vi "Nested_Case_structure.vi"() -> ()   [LabVIEW 2017]
panel:
  out "String":string
  in  "Numeric":dbl
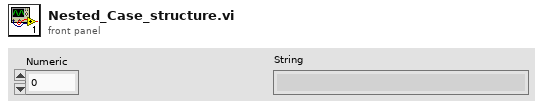
[diagram p1: front panel]
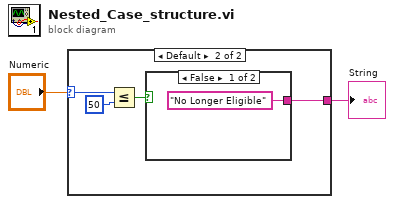
[diagram p0: block diagram]
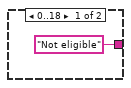
[diagram p2: hidden frame]
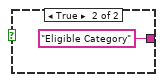
[diagram p3: hidden frame]
diagram:
  n1 = case shown="Default" "Numeric" {
    selector: "Numeric" -> [_ w7]
    tunnel: ["Not eligible" w4] -> w1
    frame 0..18 {
    }
    frame Default {
      n2 = Less Or Equal?(x=w7, y=50) -> (x <= y?=w6:bool)
      n3 = case shown="False" w6 {
        tunnel: ["No Longer Eligible" "Eligible Category"] -> w4
        frame False {
        }
        frame True {
        }
      }
    }
  }
  "String" <- w1
